vi "No Elements Saved Message--constant.vi"() -> (3 "message":string)   [LabVIEW 2020]
doc: "Message displayed to user when no elements are found for the current VI."
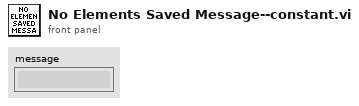
[diagram p1: front panel]
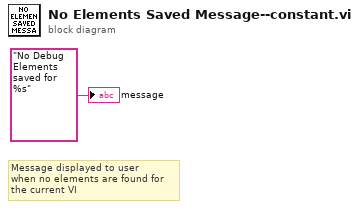
[diagram p0: block diagram]
diagram:
  # "Message displayed to user\nwhen no elements are found for\nthe current VI"
  "message" <- "No Debug Elements saved for %s" ("message")
